vi "Subpanel UI.vi"(8 "error in (no error)":errorcluster, 10 "Message Queue":refnum<queue>, 11 "Controller in":refnum<class "Generic Plugin.lvclass">) -> (0 "error out":errorcluster, 3 "Controller out":refnum<class "Generic Plugin.lvclass">)   [LabVIEW 2020, in "Generic Plugin.lvclass"]
doc: "Dynamic dispatch VI that must be overridden by all inheriting classes. It is the UI that will be inserted into subpanels so data can be displayed to the user. The class will use an internally managed message queue to communicate to it. The user should only communicate to this UI through class methods."
uses:
  Generic Plugin.lvclass
  Generic Plugin.lvclass/Generic Plugin.ctl
  Sub VIs/Message Queue/Message Cluster.ctl
  Sub VIs/Message Queue/test Message Queue.lvlib
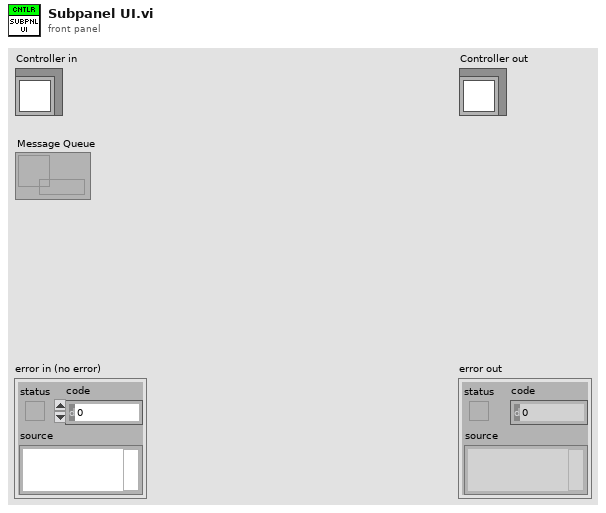
[diagram p1: front panel]
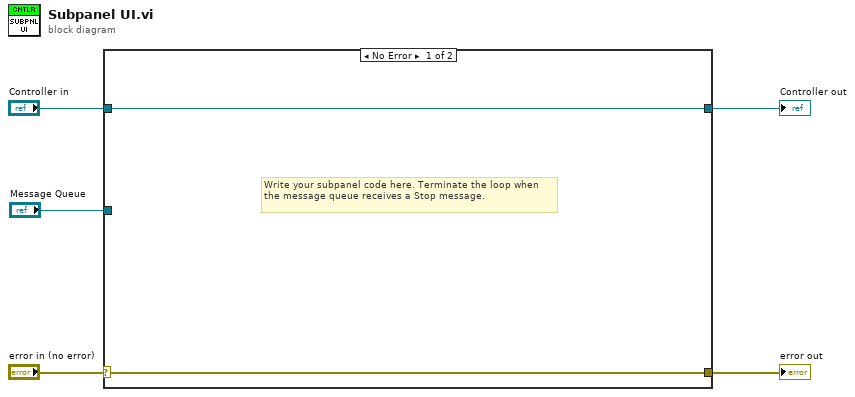
[diagram p0: block diagram]
diagram:
  n1 = case shown="No Error" "error in (no error)" {
    selector: "error in (no error)" -> [w6 w9]
    tunnel: [w6 w9] -> w4
    tunnel: [w7 w8] -> w2
    tunnel: "Controller in" -> [w7 w8]
    tunnel: "Message Queue" -> [_ _]
    frame No Error {
      # "Write your subpanel code here. Terminate the loop when the message queue receives a Stop message."
    }
    frame Error {
    }
  }
  "error out" <- w4
  "Controller out" <- w2
